vi "Script Numeric Polymorphic.vi"() -> ()   [LabVIEW 2016]
panel:
  in  "Output File":path
  in  "Array":T1(array[cluster])
  in  "Base Folder":string="C:\\Git\\SourceTree\\data-sharing-framework\\Source\\Classes\\Memory.Pointer.%s\\Methods"
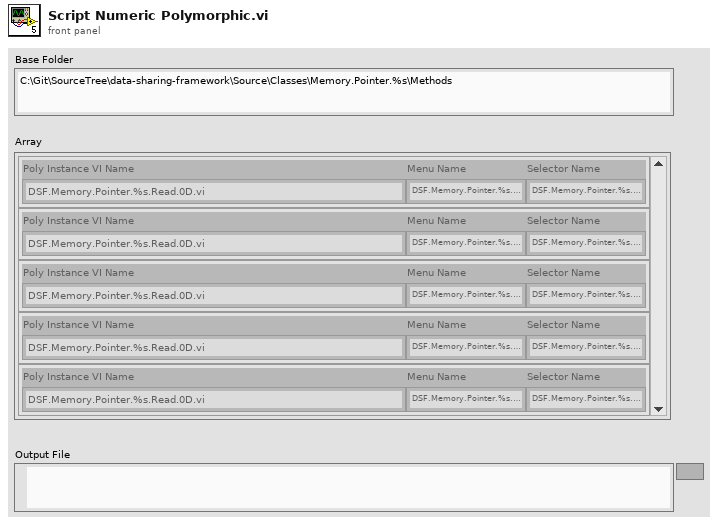
[diagram p1: front panel]
types:
  T1 = cluster{"Poly Instance VI Name":string, "Menu Name":string, "Selector Name":string}[]
  T2 = enum32{"invalid VI type", "Standard VI", "Control VI", "Global VI", "Polymorphic VI", "Configuration VI", "SubSystem", "Facade VI", "Method VI", "Statechart Diagram VI"}
  T3 = cluster{"VIPath":path, "Menu Name":string, "Selector Name":string}
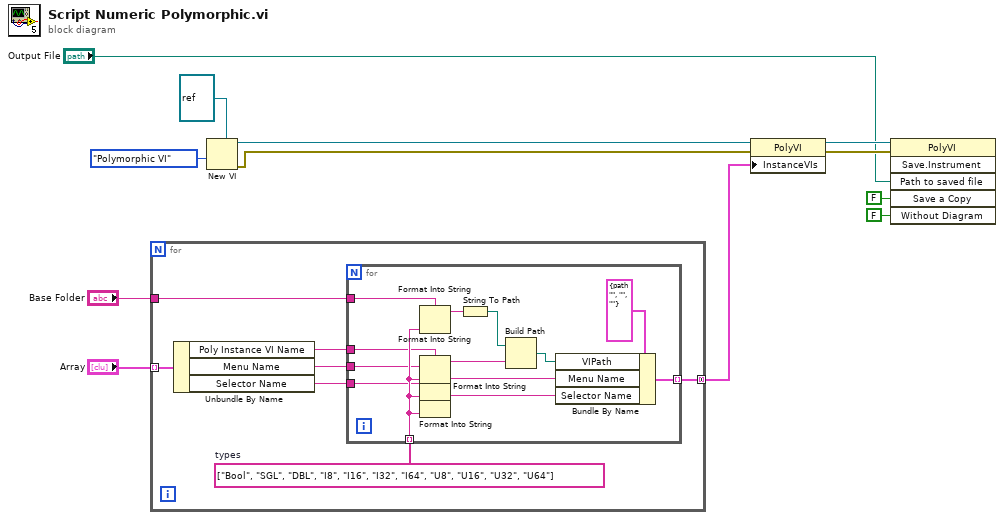
[diagram p0: block diagram]
diagram:
  n1 = for {
    tunnel: "Base Folder" -> [w19]
    tunnel: "Array" -> [w17] mode=indexing
    tunnel: [w13] -> w1 mode=concatenating
    w18 = string[] ["Bool", "SGL", "DBL", "I8", "I16", "I32", "I64", "U8", "U16", "U32", "U64"]  # types
    n2 = Unbundle By Name(w17) -> ("Poly Instance VI Name"=w16:string, "Menu Name"=w15:string, "Selector Name"=w14:string)
    n3 = for {
      tunnel: w18 -> [w26] mode=indexing
      tunnel: w19 -> [w20]
      tunnel: w16 -> [w21]
      tunnel: [w27] -> w13 mode=indexing
      tunnel: w15 -> [w22]
      tunnel: w14 -> [w23]
      n4 = Format Into String(format string=w20, w26) -> (resulting string=w32:string)  [unwired: 2 in, 1 out]
      n5 = Format Into String(format string=w21, w26) -> (resulting string=w30:string)  [unwired: 2 in, 1 out]
      n6 = Format Into String(format string=w22, w26) -> (resulting string=w25:string)  [unwired: 2 in, 1 out]
      n7 = Format Into String(format string=w23, w26) -> (resulting string=w24:string)  [unwired: 2 in, 1 out]
      n8 = String To Path(string=w32) -> (path=w31:path)
      n9 = Build Path(base path=w31, name or relative path=w30) -> (appended path=w28:path)
      n10 = Bundle By Name(cluster=T3 {"VIPath"=path "", "Menu Name"="", "Selector Name"=""}, "VIPath"=w28, "Menu Name"=w25, "Selector Name"=w24) -> (w27:T3)
    }
  }
  n11 = New VI(5:refnum<vi> refnum ("target class"), 9:T2."Polymorphic VI" ("vi type (standard vi)")) -> (0:w7:errorcluster, 3:w9:refnum<vi>)  [unwired: 5 in]
  n12 = property class="PolyVI"(reference=w9, error in=w7, "InstanceVIs"=w1) -> (reference out=w6:refnum<vi>, error out=w5:errorcluster)
  n13 = invoke class="PolyVI" method="Save.Instrument"(reference=w6, error in=w5, "Path to saved file"="Output File", "Save a Copy"=FALSE, "Without Diagram"=FALSE) -> ()  [unwired: 1 in, 6 out]
